vi "getSerial.vi"(6 "Error":bool, 7 "VISA resource name":refnum<visa-resource-name>="ASRL13::INSTR") -> (2 "Error":bool, 3 "dup VISA resource name":refnum<visa-resource-name>="ASRL13::INSTR")   [LabVIEW 2018]
panel:
  out "Serial Number":string
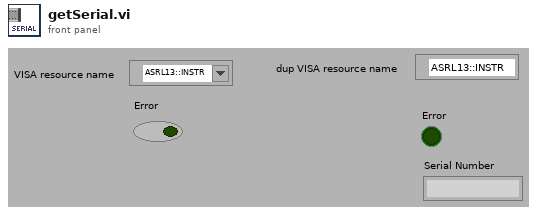
[diagram p1: front panel]
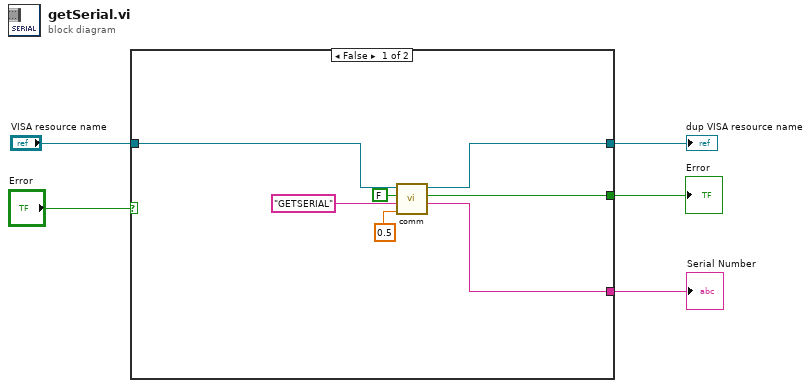
[diagram p0: block diagram]
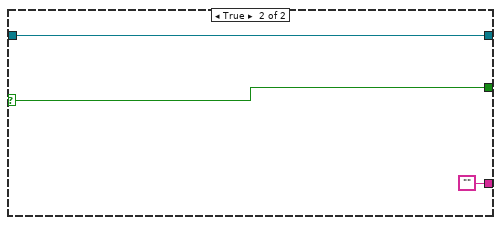
[diagram p2: hidden frame]
diagram:
  n1 = case shown="False" "Error" {
    selector: "Error" -> [_ w15]
    tunnel: "VISA resource name" -> [w12 w14]
    tunnel: [w7 w15] -> w4
    tunnel: [w11 w14] -> w3
    tunnel: [w6 ""] -> w1
    frame False {
      n2 = call "comm.vi"("Timeout (s)"=0.5, "Command"="GETSERIAL", "Error"=FALSE, "VISA resource name"=w12) -> ("Response"=w6:string, "Error"=w7:bool, "dup VISA resource name"=w11:refnum<visa-resource-name>)  [unwired: 2 in, 1 out]
    }
    frame True {
    }
  }
  "Error" <- w4
  "dup VISA resource name" <- w3
  "Serial Number" <- w1
